vi "Write Analogue.vi"(8 "error in (no error)":errorcluster, 9 "Output":bool, 10 "Channel index(0)":i32, 11 "Lambda Gen LAN in":refnum<class "Lambda Gen LAN.lvclass">) -> (0 "error out":errorcluster, 2 "Success?":bool, 3 "Lambda Gen LAN out":refnum<class "Lambda Gen LAN.lvclass">)   [LabVIEW 2025, in "Power Supply.lvlib" / "Lambda Gen LAN.lvclass"]
uses:
  Lambda Gen LAN.lvclass
  Lambda Gen LAN.lvclass/Lambda Gen LAN.ctl
  <instrlib>/TDK-Lambda GEN LAN Series/TDK-Lambda GEN LAN Series.lvlib
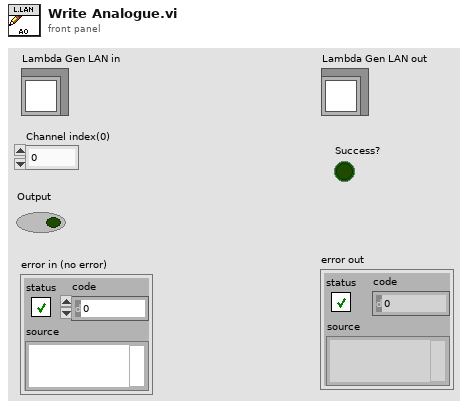
[diagram p1: front panel]
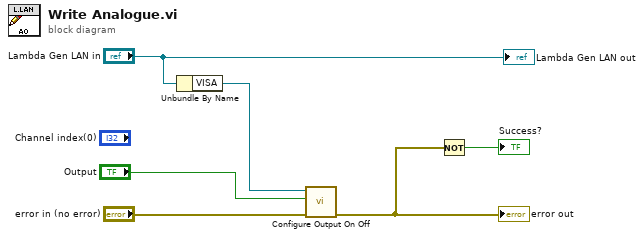
[diagram p0: block diagram]
diagram:
  n1 = Unbundle By Name("Lambda Gen LAN in") -> ("VISA"=w4:refnum<visa-resource-name>)
  n2 = call <instrlib>:"Configure Output On Off.vi"("error"="error in (no error)", "Output ON"="Output", "VISA"=w4) -> ("error out"=w2:errorcluster)  [unwired: 7 in, 1 out]
  "error out" <- w2
  n3 = Not(x=w2) -> (.not. x?=→"Success?":bool)
  "Lambda Gen LAN out" <- "Lambda Gen LAN in"
